vi "-8481 Device not Initialized--error.vi"(8 "error in":errorcluster, 11 "Instr Ident":string) -> (0 "error out":errorcluster)   [LabVIEW 2024, in "PCAN.lvlib" / "PCAN.lvclass"]
uses:
  PCAN.lvclass
  PCAN.lvclass/PCAN.ctl
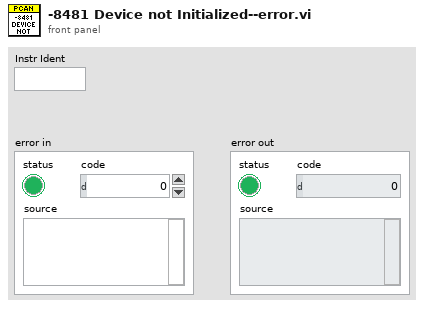
[diagram p1: front panel]
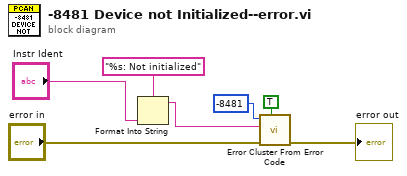
[diagram p0: block diagram]
diagram:
  n1 = Format Into String(format string="%s: Not initialized" ("error message (\"\")"), "Instr Ident") -> (resulting string=w2:string)  [unwired: 2 in, 1 out]
  n2 = call <vilib>:"Error Cluster From Error Code.vi"("show call chain? (False)"=TRUE, "error in (no error)"="error in", "error message (\"\")"=w2, "error code (0)"=-8481) -> ("error out"=→"error out":errorcluster)  [unwired: 5 in]
